vi "Day02-04_SubVI.vi"(6 "숫자형 4":dbl, 9 "숫자형 3":dbl, 10 "숫자형 2":dbl, 11 "숫자형":dbl) -> (3 "x+y":dbl)   [LabVIEW 2021]
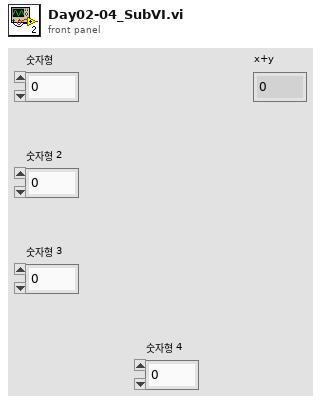
[diagram p1: front panel]
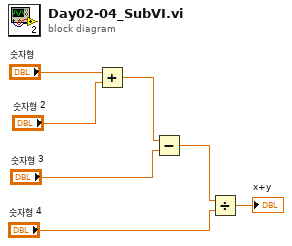
[diagram p0: block diagram]
diagram:
  n1 = Add(x="숫자형", y="숫자형 2") -> (x+y=w3:dbl)
  n2 = Subtract(x=w3, y="숫자형 3") -> (x-y=w5:dbl)
  n3 = Divide(x=w5, y="숫자형 4") -> (x/y=→"x+y":dbl)
